vi "Refresh Sub Panels.vi"(7 "Root Container":refnum<vi>, 8 "error in (no error)":errorcluster, 11 "Panels Refnums Array":T1[](array[typedef])) -> (0 "error out":errorcluster, 3 "Panels Refnums Array Out (dup)":T1[](array[typedef]))   [LabVIEW 2013, in "UI Panels.lvlib" / "Panels_XControl.xctl"]
uses:
  Panels_XControl.xctl
  Controls/References/Panel_Refnums.ctl
  Controls/Panel_Command_Enum.ctl
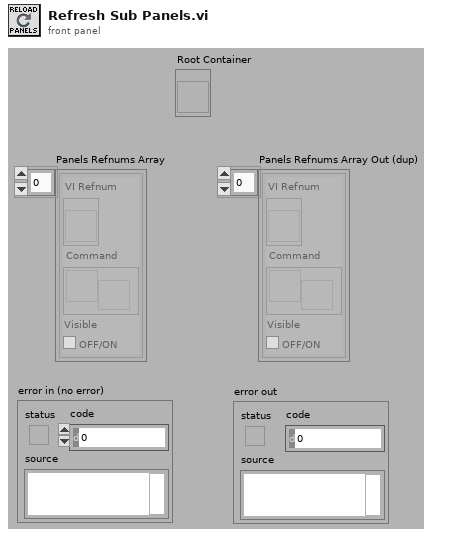
[diagram p1: front panel]
types:
  T1 = typedef "UI Panels.lvlib/Panels_XControl.xctl/Panel_Refnums.ctl" = cluster{"VI Refnum":refnum<vi>, "Command":refnum<user-event>, "Visible":bool}
  T2 = typedef "UI Panels.lvlib/Panels_XControl.xctl/Panel_Command_Enum.ctl" = enum16{"Idle", "Remove & Stop", "Add Item", "Delete Item", "Delete All", "Insert into Subpanel", "Register Menu Events", "Update Value", "Remove from Subpanel", "Set Title", "Set Menu Items", "Insert SubPanel", "Set Splitter Position", "Set Splitter Properties", "Add Menu Items"}
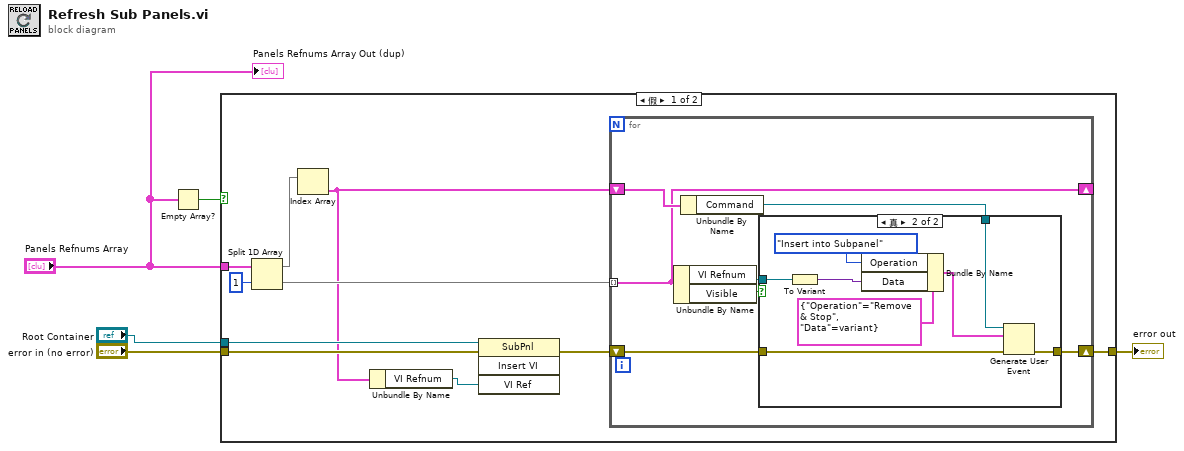
[diagram p0: block diagram]
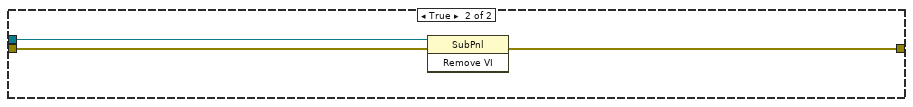
[diagram p3: hidden frame]
diagram:
  n1 = Empty Array?(array="Panels Refnums Array") -> (empty?=w2:bool)
  n2 = case shown="假" w2 {
    tunnel: "Root Container" -> [w10 w34]
    tunnel: "Panels Refnums Array" -> [w13 _]
    tunnel: "error in (no error)" -> [w9 w33]
    tunnel: [w15 w32] -> w3
    frame False {
      n3 = Split 1D Array(array=w13, index=1) -> (first subarray=w11:T1[], second subarray=w12:T1[])
      n4 = Index Array(array=w11) -> (element=w6:T1)  [unwired: 1 in]
      n5 = Unbundle By Name(w6) -> ("VI Refnum"=w7:refnum<vi>)
      n6 = invoke on="Invoke Node" class="SubPnl" method="Insert VI"(reference=w10, error in=w9, "VI Ref"=w7) -> (error out=w8:errorcluster)  [unwired: 1 in, 3 out]
      n7 = for {
        tunnel: w12 -> [w19] mode=indexing
        shift-right: [w21] -> w15
        shift-left: w8 -> [w22]
        shift-right: [w19] -> _
        shift-left: w6 -> [w20]
        n8 = Unbundle By Name(w19) -> ("VI Refnum"=w17:refnum<vi>, "Visible"=w16:bool)
        n9 = Unbundle By Name(w20) -> ("Command"=w18:refnum<user-event>)
        n10 = case shown="真" w16 {
          tunnel: w18 -> [_ w28]
          tunnel: [w23 w27] -> w21
          tunnel: w17 -> [_ w30]
          tunnel: w22 -> [w23 w25]
          frame False {
          }
          frame True {
            n11 = To Variant(anything=w30) -> (Variant=w29:variant)
            n12 = Bundle By Name(cluster=cluster{"Operation":T2, "Data":variant} {"Operation"=enum."Remove & Stop", "Data"=variant} ("Item_Command"), "Operation"=Panel_Command_Enum."Insert into Subpanel", "Data"=w29) -> (w26:cluster{"Operation":T2, "Data":variant})
            n13 = Generate User Event(user event=w28, event data cluster=w26, error in=w25) -> (error out=w27:errorcluster)  [unwired: 1 in, 1 out]
          }
        }
      }
    }
    frame True {
      n14 = invoke on="Invoke Node" class="SubPnl" method="Remove VI"(reference=w34, error in=w33) -> (error out=w32:errorcluster)  [unwired: 1 in, 2 out]
    }
  }
  "error out" <- w3
  "Panels Refnums Array Out (dup)" <- "Panels Refnums Array"
